vi "Dialog_DeleteConfirm.vi"() -> (3 "OK?":bool)   [LabVIEW 2012]
doc: "SciScan 1.2 160622"
panel:
  in  "Cancel Button":bool
  in  "OK Button":bool
  # "Confirmation Required!"
  # "This will delete the selected position. Are you sure?"
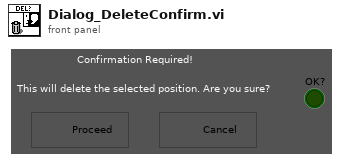
[diagram p1: front panel]
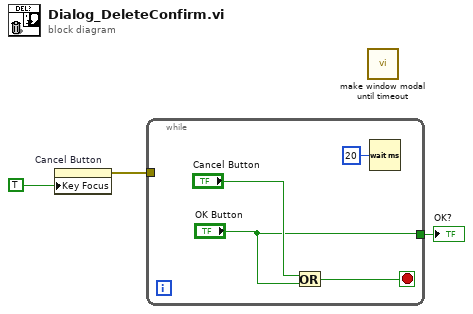
[diagram p0: block diagram]
diagram:
  n1 = property on="Cancel Button" class="Bool"("Key Focus"=TRUE) -> (error out=w1:errorcluster)  [unwired: 2 in, 1 out]
  n2 = while {
    tunnel: ["OK Button"] -> w3
    tunnel: w1 -> [_]
    stop <- w5 stop-if-true
    n3 = Or(x="Cancel Button", y="OK Button") -> (x .or. y?=w5:bool)
    n4 = Wait (ms)(milliseconds to wait=u32 20) -> ()  [unwired: 1 out]
  }
  "OK?" <- w3
  n5 = call "make window modal until timeout.vi"() -> ()  [unwired: 12 in]
